vi "2_Data_Convert_SubVI.vi"(1 "hata sim":bool, 2 "data in":string) -> (0 "tx write":string)   [LabVIEW 2024]
panel:
  out "subarray":u8[](array[numeric]) format="%02x"
  out "size(s) 2":i32
  out "output array":u8[](array[numeric]) format="%02x"
  out "size(s)":i32
  out "concatenated string":string
  out "sum":u16
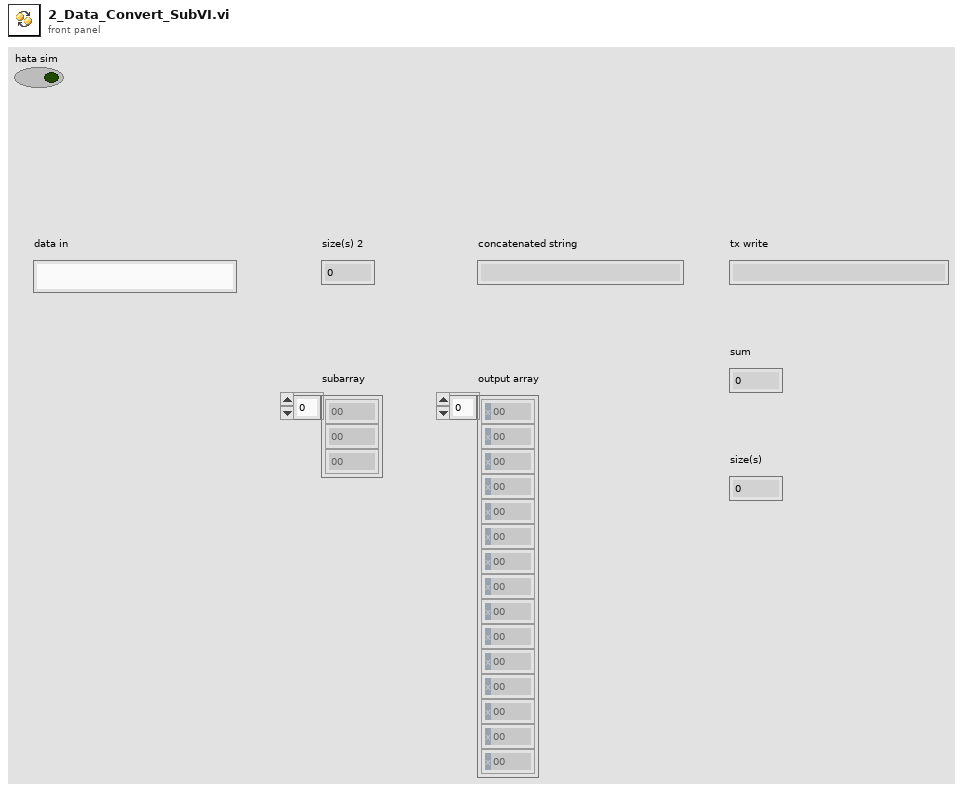
[diagram p1: front panel]
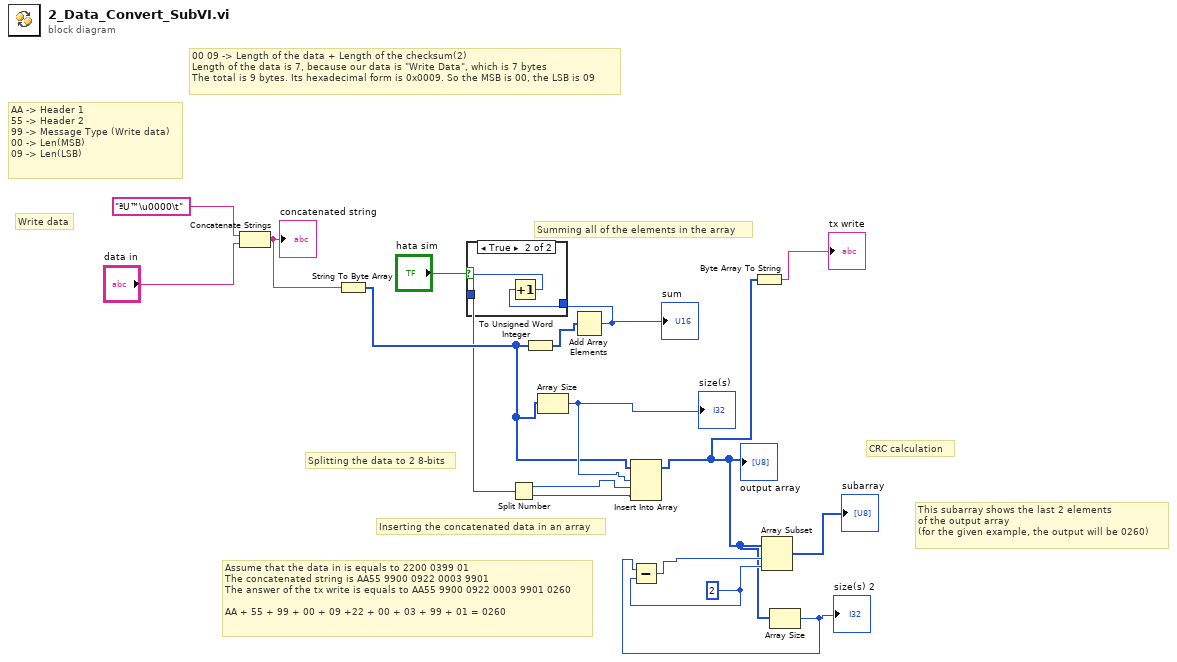
[diagram p0: block diagram]
diagram:
  w17 = 2 ("length")
  # "CRC calculation"
  # "Write data"
  # "This subarray shows the last 2 elements\nof the output array\n(for the given example, the output will be 0260)"
  # "Assume that the data in is equals to 2200 0399 01\nThe concatenated string is AA55 9900 0922 0003 9901 \nThe answer of the tx write is equals to AA55 9900 0922 0003 9901 0260 \n\nAA + 55 + 99 + 00 + 09 +22 + 00 + 03 + 99 + 01 = 0260"
  # "Inserting the concatenated data in an array"
  # "Splitting the data to 2 8-bits"
  # "Summing all of the elements in the array"
  # "00 09 -> Length of the data + Length of the checksum(2)\nLength of the data is 7, because our data is \"Write Data\", which is 7 bytes\nThe total is 9 bytes. Its hexadecimal form is 0x0009. So the MSB is 00, the LSB is 09"
  # "AA -> Header 1\n55 -> Header 2\n99 -> Message Type (Write data)\n00 -> Len(MSB)\n09 -> Len(LSB)"
  n1 = Concatenate Strings "Concatenate Strings"("ªU™\u0000\t", "data in") -> (w7:string)
  "concatenated string" <- w7
  n2 = String To Byte Array(string=w7) -> (unsigned byte array=w8:u8[])
  n3 = To Unsigned Word Integer(number=w8) -> (unsigned 16bit integer=w4:u16[])
  n4 = Array Size(array=w8) -> (size(s)=w9:i32)
  "size(s)" <- w9
  n5 = Add Array Elements(numeric array=w4) -> (sum=w3:u16)
  "sum" <- w3
  n6 = case shown="True" "hata sim" {
    tunnel: w3 -> [w18 w20]
    tunnel: [w18 w19] -> w2
    frame False {
    }
    frame True {
      n7 = Increment(x=w20) -> (x+1=w19:u16)
    }
  }
  n8 = Split Number(x=w2) -> (hi(x)=w10:u8, lo(x)=w11:u8)
  n9 = Insert Into Array "Insert Into Array"(array=w8, index=w9, new element #1=w10, new element #2=w11) -> (w13:u8[])
  "output array" <- w13
  n10 = Byte Array To String(unsigned byte array=w13) -> (string=→"tx write":string)
  n11 = Array Size(array=w13) -> (size(s)=w15:i32)
  "size(s) 2" <- w15
  n12 = Subtract(x=w15, y=w17) -> (x-y=w16:i32)
  n13 = Array Subset "Array Subset"(array=w13, index=w16, length=w17) -> (→"subarray":u8[])
